vi "Write GUI Events.vi"(8 "error in (no error)":errorcluster, 10 "GUI Events":cluster{"Stop":refnum<user-event>}, 11 "CS++Scope in":refnum<class "CS++Scope.lvclass">) -> (0 "error out":errorcluster, 3 "CS++Scope out":refnum<class "CS++Scope.lvclass">)   [LabVIEW 2014, in "CS++Scope.lvlib" / "CS++Scope.lvclass"]
uses:
  CS++Scope.lvclass
  CS++Scope.lvclass/CS++Scope.ctl
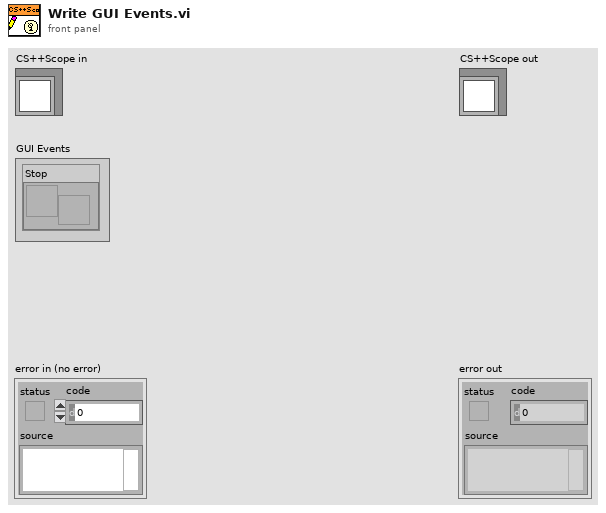
[diagram p1: front panel]
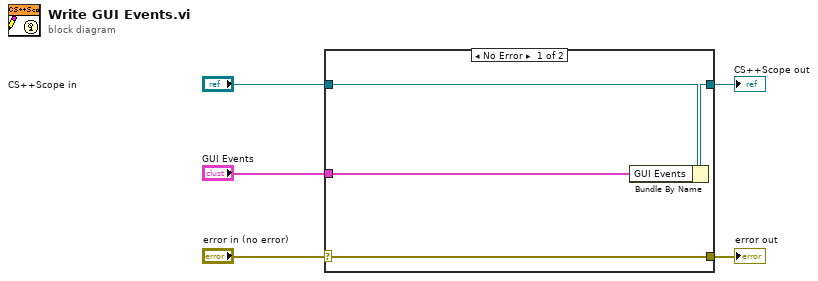
[diagram p0: block diagram]
diagram:
  n1 = case shown="No Error" "error in (no error)" {
    selector: "error in (no error)" -> [w9 w10]
    tunnel: [w9 w10] -> w4
    tunnel: [w7 w11] -> w2
    tunnel: "CS++Scope in" -> [w8 w11]
    tunnel: "GUI Events" -> [w6 _]
    frame No Error {
      n2 = Bundle By Name(cluster=w8, "GUI Events"=w6) -> (w7:refnum<class "CS++Scope.lvclass">)
    }
    frame Error {
    }
  }
  "error out" <- w4
  "CS++Scope out" <- w2
